vi "RT Main v0.96.vi"() -> ()   [LabVIEW 2017]
doc: "Changelog:\n\nv0.9:\n- Autocycle"
uses:
  Controls/Auto Delays.ctl
  support/Controls/All Inputs.ctl
  support/Controls/Index Details.ctl
  support/Controls/Auto Stats.ctl
  Controls/Auto Times.ctl
  Global Variables/RT GV.vi
  support/Message Queue/Enqueue Message (Single).vi
  Global Variables/FPGA GV.vi
  <vilib>/Utility/error.llb/Error Cluster From Error Code.vi
  <vilib>/rvi/errors/niLvFpgaAdjustHostInterfaceError.vi
  Global Variables/Network Globals.vi
  <vilib>/FPGAPlugInAG/Dynamic/niLvFpga_Close_Dynamic.vi
  <vilib>/rvi/interface/nirviReadWriteControl/nirviReadWriteControl.xnode
  Controls/FPGA Ref.ctl
  <vilib>/rvi/interface/nirviCloseFPGA/nirviCloseFPGA.xnode
  support/Message Queue/Message Queue.lvlib
  NiFpgaLv.dll
  <vilib>/rvi/interface/Simulation/niFpgaSimulationCallBeginRW.vi
panel:
  in  "Auto Para":T1={"Agitator Delays"=[250, 350], "TF Delays"=[700, 800, 2], "Insertion Delays"=[100, 500], "Cutting Delays"=[300, 300, 100], "PF Delays"=[250, 30000], "Measur. Delays"=[500.0, 188.9, 1.0], "Reject Delays"=[500], "BF Delays"=[1000, 1000]}
  in  "Counts in":cluster{"OutputCount":u32, "RejectCount":u32}
  in  "Stop Button 4":bool
  out "error out":errorcluster
  out "Wrong Message":string
  in  "Stop Button":bool
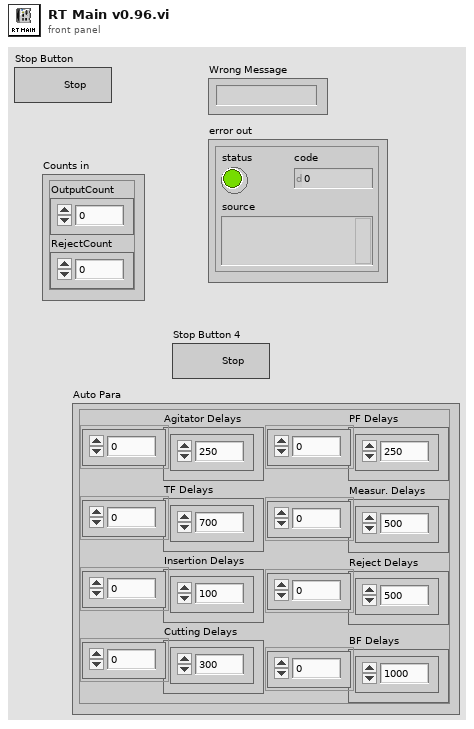
[diagram p1: front panel]
types:
  T1 = typedef "Auto Delays.ctl" = cluster{"Agitator Delays":u32[], "TF Delays":u32[], "Insertion Delays":u32[], "Cutting Delays":u32[], "PF Delays":u32[], "Measur. Delays":dbl[], "Reject Delays":u32[], "BF Delays":u32[]}
  T2 = typedef "FPGA Ref.ctl" = refnum<k20>
  T3 = cluster{"TL_Red":bool, "TL_Orange":bool, "TL_Green":bool, "TL_Buzzer":bool, "SOL_Index_Rotary_CW":bool, "SOL_Index_CNVR_Rotary_CCW":bool, "SOL_Index_CNVR_Stopper_Rear":bool, "SOL_Index_CNVR_Output _Separator _Rear":bool, "Bowl  Feeder_ ON":bool, "Pump_CNVR_Motor _ON":bool, "SOL_Gating_CYL_Rear":bool, "SOL_Tube_Feed_Agitatator":bool, "SOL_Tube_Feed_Gating_CYL":bool, "SOL_Insertion _CYL":bool, "SOL_Insertion_Clamp_CYL":bool, "SOL_Cutting_CYL":bool, "SOL_Cutting_Clamp_CYL":bool, "SOL_Insertion_Air_Nozzle":bool, "SOL_Measurement_CYL":bool, "SOL_Measure_Clamp_CYL":bool, "SOL_Rejection CYL_1":bool, "SOL_Rejection CYL_2":bool, "SOL_Rejection CYL_3":bool, "SOL_Rejection CYL_4":bool, "DO1.24":bool, "DO1.25":bool, "DO1.26":bool, "DO1.27":bool, "DO1.28":bool, "DO1.29":bool, "DO1.30":bool, "DO1.31":bool}
  T4 = typedef "All Inputs.ctl" = cluster{"DI 1":cluster{"Machine_ON":bool, "E_stop ":bool, "SW_Pressure":bool, "SW_Start ":bool, "SW_Reset":bool, "SW_Stop":bool, "SW_Door":bool, "RS_Index_Rotary_CW":bool, "RS_Index_Rotary_CCW":bool, "RS_Index_Stopper _Rear":bool, "RS_Index_Output_Separator_Rear":bool, "PES_Index_Pallet_Sensor":bool, "PES_Index_Output_Part Sensor":bool, "ICS_BF_Low_Level_1":bool, "ICS_BF_Low_Level_2":bool, "ICS_BF_Pump_CNVR_Full_1":bool, "ICS_BF_Pump_CNVR_Full_2":bool, "ICS_BF_Pump_CNVR_Full_3":bool, "ICS_BF_Pump_CNVR_Full_4":bool, "PES_PC_Pump Presence_1":bool, "PES_PC_Pump Presence_2":bool, "PES_PC_Pump Presence_3":bool, "PES_PC_Pump Presence_4":bool, "RS_PC_Gating_Front":bool, "PES_Pump_Interference":bool, "PES_TF_Low_Level":bool, "PES_Tube Presence_1":bool, "PES_Tube Presence_2":bool, "PES_Tube Presence_3":bool, "PES_Tube Presence_4":bool, "DI1.30":bool, "DI1.31":bool}, "DI 2":cluster{"RS_Agitatator_1_Rear ":bool, "RS_Agitatator_2_Rear ":bool, "RS_TF_Gating CYL_Rear":bool, "RS_Insertion_1_Rear":bool, "RS_Insertion_1_Front":bool, "RS_Insertion _2_Rear":bool, "RS_Insertion _2_Front":bool, "RS_Insertion _3_Rear":bool, "RS_Insertion _3_Front":bool, "RS_Insertion _4_Rear":bool, "RS_Insertion _4_Front":bool, "RS_Insertion_Clamp_Rear":bool, "RS_Cutting_Rear":bool, "RS_Cutting_Clamp _Rear":bool, "RS_Measurement_1_Rear":bool, "RS_Measurement_2_Rear":bool, "RS_Measurement_3_Rear":bool, "RS_Measurement_4_Rear":bool, "RS_Measure_Clamp_Rear":bool, "RS_Rejection_1_Rear":bool, "RS_Rejection_2_Rear":bool, "RS_Rejection_3_Rear":bool, "RS_Rejection_4_Rear":bool, "DI2.23":bool, "DI2.24":bool, "DI2.25":bool, "DI2.26":bool, "DI2.27":bool, "DI2.28":bool, "DI2.29":bool, "DI2.30":bool, "DI2.31":bool}, "IAS 1":dbl, "IAS 2":dbl, "IAS 3":dbl, "IAS 4":dbl, "DO 1":cluster{"TL_Red":bool, "TL_Orange":bool, "TL_Green":bool, "TL_Buzzer":bool, "SOL_Index_Rotary_CW":bool, "SOL_Index_CNVR_Rotary_CCW":bool, "SOL_Index_CNVR_Stopper_Rear":bool, "SOL_Index_CNVR_Output _Separator _Rear":bool, "Bowl  Feeder_ ON 1":bool, "Pump_CNVR_Motor _ON":bool, "SOL_PC_Gating_CYL_Rear":bool, "SOL_Tube_Feed_Agitatator":bool, "SOL_Tube_Feed_Gating_CYL":bool, "SOL_Insertion _CYL":bool, "SOL_Insertion_Clamp_CYL":bool, "SOL_Cutting_CYL":bool, "SOL_Cutting_Clamp_CYL":bool, "SOL_Insertion_Air_Nozzle":bool, "SOL_Measurement_CYL":bool, "DO1.19":bool, "SOL_Rejection CYL_1":bool, "SOL_Rejection CYL_2":bool, "SOL_Rejection CYL_3":bool, "SOL_Rejection CYL_4":bool, "Bowl  Feeder_ ON 2":bool, "SOL_BF_BlowerON":bool, "SOL_BF1_Track1":bool, "SOL_BF1_Track2":bool, "SOL_BF2_Track1":bool, "SOL_BF2_Track2":bool, "DO1.30":bool, "DO1.31":bool}}
  T5 = typedef "Index Details.ctl" = cluster{"Time (ms)":u32, "Waveform Graph":i16[]}
  T6 = cluster{T1, "Reject Pallets":cluster{"Reject 1":bool, "Reject 2":bool, "Reject 3":bool, "Reject 4":bool}}
  T7 = typedef "Auto Stats.ctl" = cluster{"Time":timestamp, "OEE":cluster{"AVL":dbl, "PRF":dbl, "QUA":dbl, "OEE":dbl}, "Auto Times":T8, "Counts out":cluster{"OutputCount":u32, "RejectCount":u32}, "Measurements":cluster{"1":dbl, "2":dbl, "3":dbl, "4":dbl}, "Outputs":cluster{"OutputCount":u32, "Numeric Control":u32}}
  T8 = typedef "Auto Times.ctl" = cluster{"Index Time":u32, "TF Time":u32, "Insertion Time":u32, "Cutting Time":u32, "PF Time":u32, "Meas. Time":u32, "Reject Time":u32}
  T9 = cluster{string, dbl, "Counts in":cluster{"OutputCount":u32, "RejectCount":u32}, "Auto Para":T1}
  T10 = cluster{"TL_Red":bool, "TL_Orange":bool, "TL_Green":bool, "TL_Buzzer":bool, "SOL_Index_Rotary_CW":bool, "SOL_Index_CNVR_Rotary_CCW":bool, "SOL_Index_CNVR_Stopper_Rear":bool, "SOL_Index_CNVR_Output _Separator _Rear":bool, "Bowl Feeder_ ON1":bool, "Pump_CNVR_Motor _ON":bool, "SOL_PC_Gating_CYL_Rear":bool, "SOL_Tube_Feed_Agitatator":bool, "SOL_Tube_Feed_Gating_CYL":bool, "SOL_Insertion _CYL":bool, "SOL_Insertion_Clamp_CYL":bool, "SOL_Cutting_CYL":bool, "SOL_Cutting_Clamp_CYL":bool, "SOL_Insertion_Air_Nozzle":bool, "SOL_Measurement_CYL":bool, "DO1.19":bool, "SOL_Rejection CYL_1":bool, "SOL_Rejection CYL_2":bool, "SOL_Rejection CYL_3":bool, "SOL_Rejection CYL_4":bool, "Bowl Feeder_ON2":bool, "SOL_BF_BlowerON":bool, "SOL_BF1_Track1":bool, "SOL_BF1_Track2":bool, "SOL_BF2_Track1":bool, "SOL_BF2_Track2":bool, "DO1.30":bool, "DO1.31":bool}
  T11 = cluster{"Machine_ON":bool, "E_stop ":bool, "SW_Pressure":bool, "SW_Start ":bool, "SW_Reset":bool, "SW_Stop":bool, "SW_Door":bool, "RS_Index_Rotary_CW":bool, "RS_Index_Rotary_CCW":bool, "RS_Index_Stopper _Rear":bool, "RS_Index_Output_Separator_Rear":bool, "PES_Index_Pallet_Sensor":bool, "PES_Index_Output_Part Sensor":bool, "ICS_BF_Low_Level_1":bool, "ICS_BF_Low_Level_2":bool, "ICS_BF_Pump_CNVR_Full_1":bool, "ICS_BF_Pump_CNVR_Full_2":bool, "ICS_BF_Pump_CNVR_Full_3":bool, "ICS_BF_Pump_CNVR_Full_4":bool, "PES_PC_Pump Presence_1":bool, "PES_PC_Pump Presence_2":bool, "PES_PC_Pump Presence_3":bool, "PES_PC_Pump Presence_4":bool, "RS_PC_Gating_Front":bool, "PES_Pump_Interference":bool, "PES_TF_Low_Level":bool, "PES_Tube Presence_1":bool, "PES_Tube Presence_2":bool, "PES_Tube Presence_3":bool, "PES_Tube Presence_4":bool, "DI1.30":bool, "DI1.31":bool}
  T12 = cluster{"RS_Agitatator_1_Rear ":bool, "RS_Agitatator_2_Rear ":bool, "RS_TF_Gating CYL_Rear":bool, "RS_Insertion_1_Rear":bool, "RS_Insertion_1_Front":bool, "RS_Insertion _2_Rear":bool, "RS_Insertion _2_Front":bool, "RS_Insertion _3_Rear":bool, "RS_Insertion _3_Front":bool, "RS_Insertion _4_Rear":bool, "RS_Insertion _4_Front":bool, "RS_Insertion_Clamp_Rear":bool, "RS_Cutting_Rear":bool, "RS_Cutting_Clamp _Rear":bool, "RS_Measurement_1_Rear":bool, "RS_Measurement_2_Rear":bool, "RS_Measurement_3_Rear":bool, "RS_Measurement_4_Rear":bool, "DI2.18":bool, "RS_Rejection_1_Rear":bool, "RS_Rejection_2_Rear":bool, "RS_Rejection_3_Rear":bool, "RS_Rejection_4_Rear":bool, "DI2.23":bool, "DI2.24":bool, "DI2.25":bool, "DI2.26":bool, "DI2.27":bool, "DI2.28":bool, "DI2.29":bool, "DI2.30":bool, "DI2.31":bool}
  T13 = cluster{"Array":string[][], "Machine Status":string}
  T14 = cluster{"Measurements":cluster{"1":dbl, "2":dbl, "3":dbl, "4":dbl}, "Reject Pallets":cluster{"Reject 1":bool, "Reject 2":bool, "Reject 3":bool, "Reject 4":bool}}
  T15 = cluster{"Auto Times":T8, "Results":cluster{"Measurements":cluster{"1":dbl, "2":dbl, "3":dbl, "4":dbl}, "Reject Pallets":cluster{"Reject 1":bool, "Reject 2":bool, "Reject 3":bool, "Reject 4":bool}}, "OutputCount":u32, "error out":errorcluster}
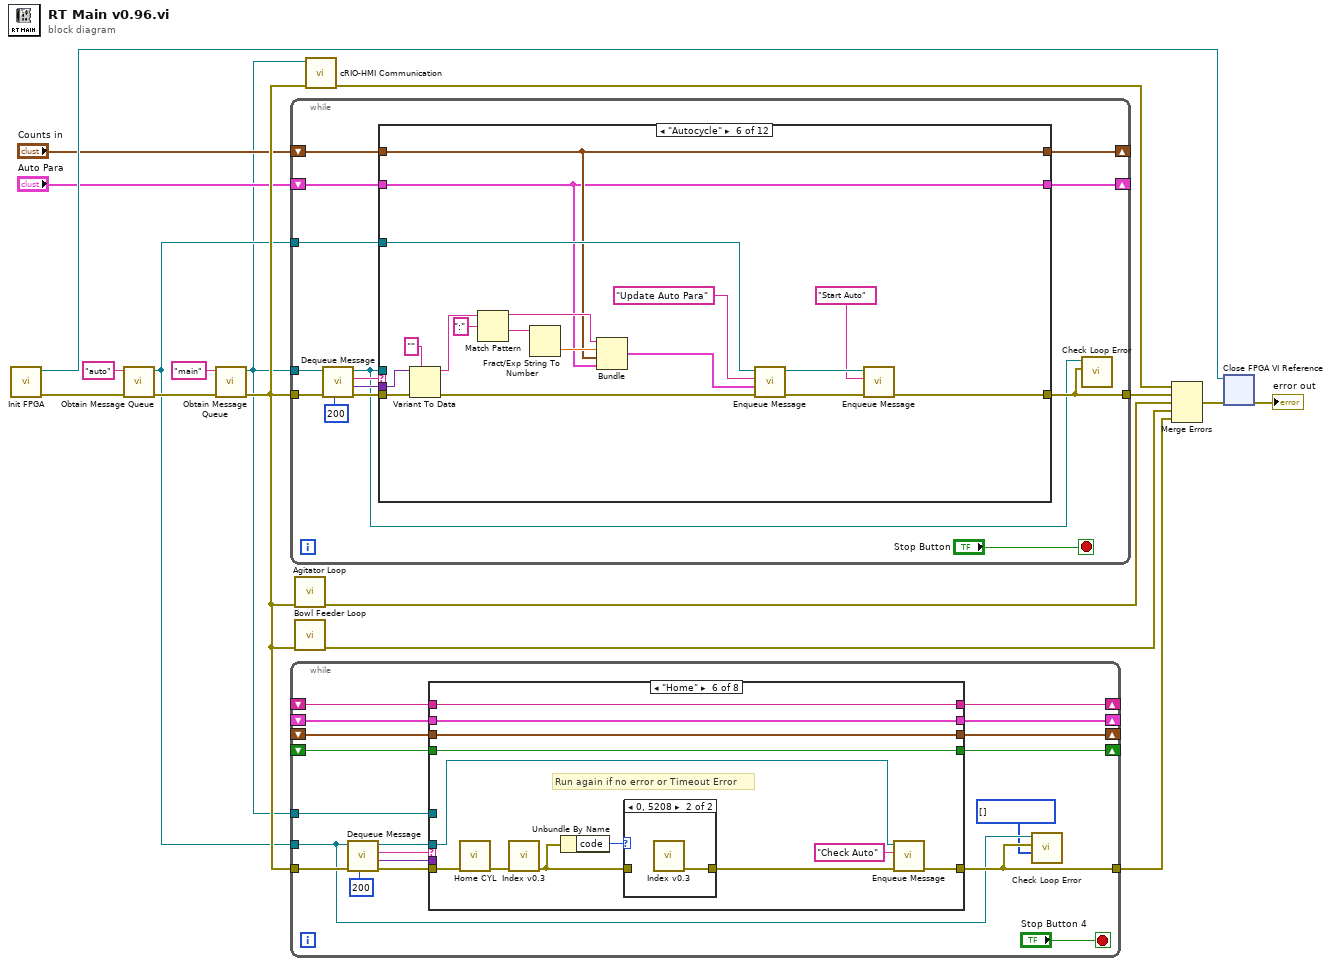
[diagram p0: block diagram]
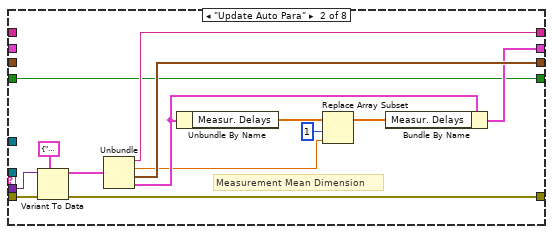
[diagram p3: hidden frame]
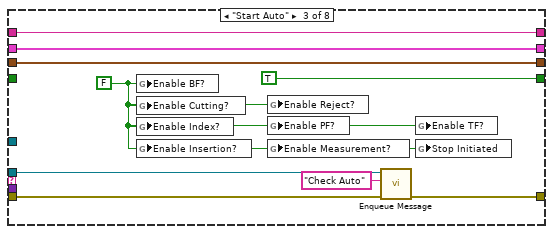
[diagram p4: hidden frame]
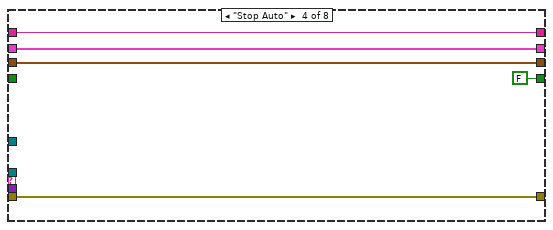
[diagram p5: hidden frame]
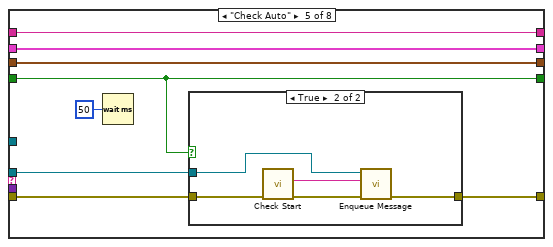
[diagram p6: hidden frame]
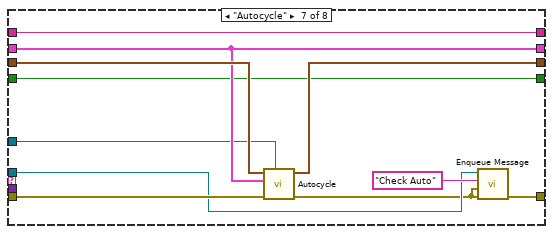
[diagram p9: hidden frame]
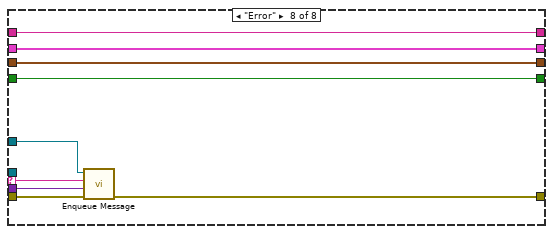
[diagram p10: hidden frame]
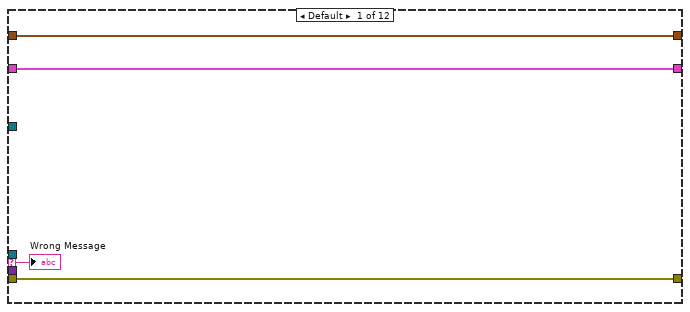
[diagram p11: hidden frame]
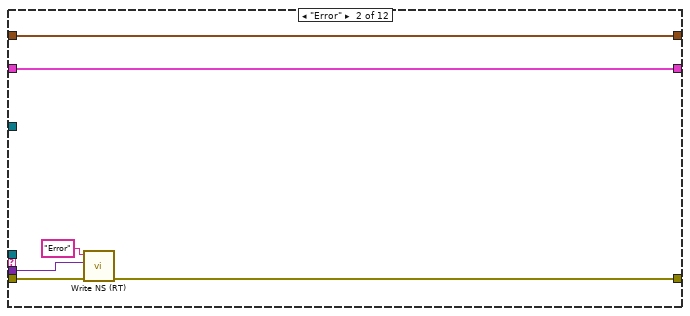
[diagram p12: hidden frame]
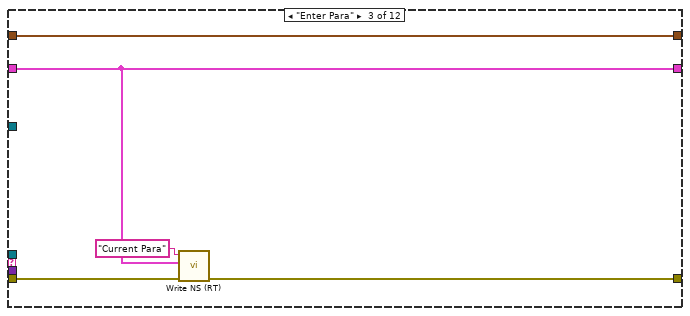
[diagram p13: hidden frame]
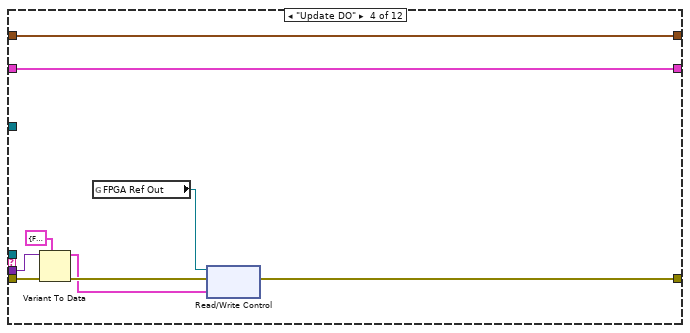
[diagram p14: hidden frame]
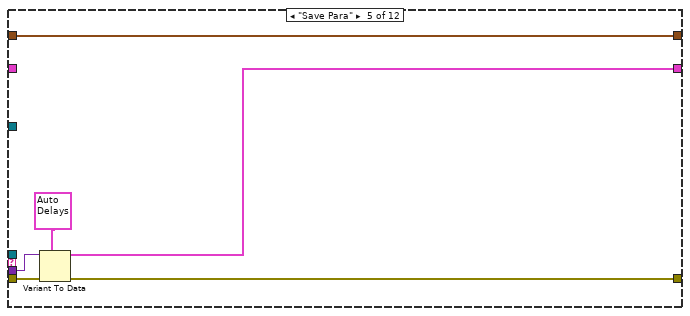
[diagram p15: hidden frame]
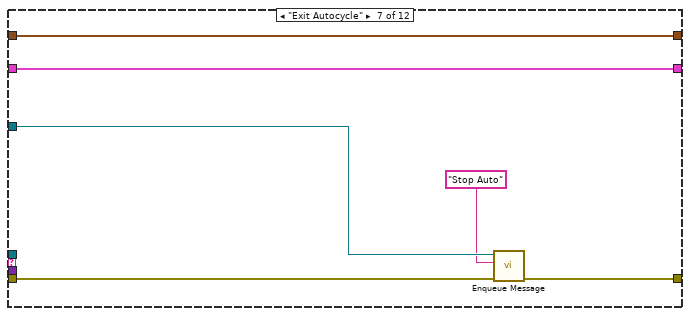
[diagram p16: hidden frame]
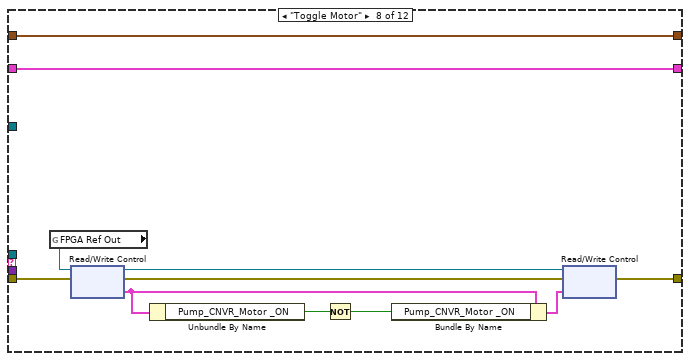
[diagram p17: hidden frame]
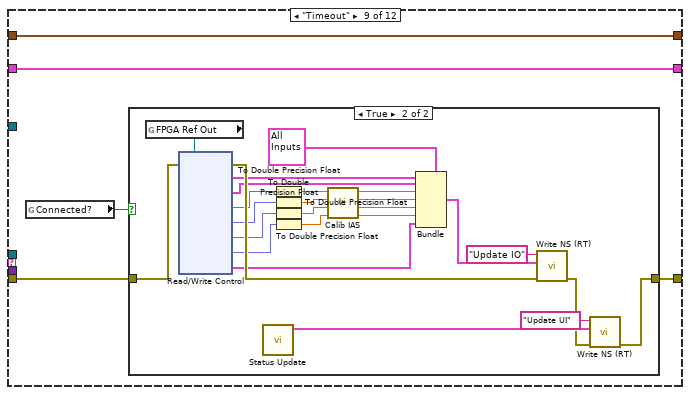
[diagram p18: hidden frame]
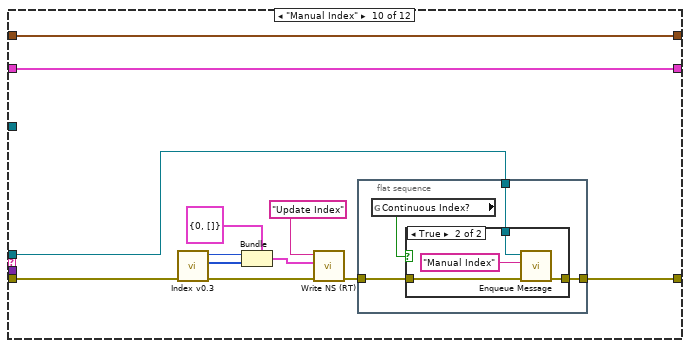
[diagram p20: hidden frame]
diagram:
  n1 = call "Init FPGA.vi"() -> ("error out"=w6:errorcluster, "FPGA Ref Out"=w11:T2)  [unwired: 10 in]
  n2 = call "Obtain Message Queue.vi"("error in (no error)"=w6, "name"="auto") -> ("error out"=w5:errorcluster, "Message Queue"=w2:refnum<queue>)  [unwired: 8 in]
  n3 = call "Obtain Message Queue.vi"("error in (no error)"=w5, "name"="main") -> ("error out"=w10:errorcluster, "Message Queue"=w1:refnum<queue>)  [unwired: 8 in]
  n4 = while {
    tunnel: w10 -> [w30]
    tunnel: w1 -> [w29]
    tunnel: [w25] -> w17
    tunnel: w2 -> [w22]
    shift-right: [w19] -> _
    shift-left: "Auto Para" -> [w20]
    shift-right: [w18] -> _
    shift-left: "Counts in" -> [w21]
    stop <- "Stop Button" stop-if-true
    n5 = call "Dequeue Message.vi"("timeout"=200, "error in (no error)"=w30, "Message Queue"=w29) -> ("error out"=w28:errorcluster, "Message Data"=w26:variant, "Message"=w27:string, "dup Message Queue"=w24:refnum<queue>)  [unwired: 5 in]
    n6 = case shown="\"Autocycle\"" w27 {
      selector: w27 -> [w35 _ _ _ _ _ _ _ _ _ _ _]
      tunnel: w28 -> [w34 w39 w46 w55 w61 w79 w85 w95 w100 w139 w166 w176]
      tunnel: w24 -> [_ _ _ _ _ _ _ _ _ w131 _ _]
      tunnel: w26 -> [_ w37 _ w54 w60 w78 _ _ _ _ w165 w175]
      tunnel: [w34 w38 w45 w50 w59 w64 w81 w93 w101 w132 w161 w172] -> w25
      tunnel: w22 -> [_ _ _ _ _ w71 w84 _ _ _ _ _]
      tunnel: w21 -> [w33 w41 w43 w48 w58 w68 w83 w87 w98 w128 w152 w171]
      tunnel: w20 -> [w32 w40 w42 w47 _ w67 w82 w86 w97 w129 w151 w170]
      tunnel: [w32 w40 w42 w47 w57 w67 w82 w86 w97 w129 w151 w170] -> w19
      tunnel: [w33 w41 w43 w48 w58 w68 w83 w87 w98 w128 w152 w171] -> w18
      frame Default {
        "Wrong Message" <- w35
      }
      frame "Error" {
        n7 = call "Write NS (RT).vi"("error in (no error)"=w39, "Message Data"=w37, "Message"="Error") -> ("error out"=w38:errorcluster)  [unwired: 8 in]
      }
      frame "Enter Para" {
        n8 = call "Write NS (RT).vi"("error in (no error)"=w46, "Message Data"=w42, "Message"="Current Para") -> ("error out"=w45:errorcluster)  [unwired: 8 in]
      }
      frame "Update DO" {
        n9 = Variant To Data(error in=w55, type=T3 {"TL_Red"=FALSE, "TL_Orange"=FALSE, "TL_Green"=FALSE, "TL_Buzzer"=FALSE, "SOL_Index_Rotary_CW"=FALSE, "SOL_Index_CNVR_Rotary_CCW"=FALSE, "SOL_Index_CNVR_Stopper_Rear"=FALSE, "SOL_Index_CNVR_Output _Separator _Rear"=FALSE, "Bowl  Feeder_ ON"=FALSE, "Pump_CNVR_Motor _ON"=FALSE, "SOL_Gating_CYL_Rear"=FALSE, "SOL_Tube_Feed_Agitatator"=FALSE, "SOL_Tube_Feed_Gating_CYL"=FALSE, "SOL_Insertion _CYL"=FALSE, "SOL_Insertion_Clamp_CYL"=FALSE, "SOL_Cutting_CYL"=FALSE, "SOL_Cutting_Clamp_CYL"=FALSE, "SOL_Insertion_Air_Nozzle"=FALSE, "SOL_Measurement_CYL"=FALSE, "SOL_Measure_Clamp_CYL"=FALSE, "SOL_Rejection CYL_1"=FALSE, "SOL_Rejection CYL_2"=FALSE, "SOL_Rejection CYL_3"=FALSE, "SOL_Rejection CYL_4"=FALSE, "DO1.24"=FALSE, "DO1.25"=FALSE, "DO1.26"=FALSE, "DO1.27"=FALSE, "DO1.28"=FALSE, "DO1.29"=FALSE, "DO1.30"=FALSE, "DO1.31"=FALSE} ("DO 1"), Variant=w54) -> (data=w49:T3, error out=w51:errorcluster)
        n10 = global read "FPGA GV.vi" "FPGA Ref Out"() -> (w52:T2)
        n11 = xnode "Read/Write Control"("FPGA VI Reference In"=w52, "error in"=w51, "DO 1"=w49) -> ("error out"=w50:errorcluster)  [unwired: 1 out]
      }
      frame "Save Para" {
        n12 = Variant To Data(error in=w61, type=T1 {"Agitator Delays"=[700, 250], "TF Delays"=[700, 800, 2], "Insertion Delays"=[100, 500], "Cutting Delays"=[300, 300, 100], "PF Delays"=[250, 30000], "Measur. Delays"=[500.0, 188.9, 1.0], "Reject Delays"=[500], "BF Delays"=[1000, 1000]} ("Auto Para"), Variant=w60) -> (data=w57:T1, error out=w59:errorcluster)
      }
      frame "Autocycle" {
        n13 = Variant To Data(error in=w79, type="", Variant=w78) -> (data=w74:string, error out=w72:errorcluster)
        n14 = Match Pattern(string=w74, regular expression=":") -> (before substring=w70:string, after substring=w75:string)  [unwired: 1 in, 2 out]
        n15 = Fract/Exp String To Number(string=w75) -> (number=w69:dbl)  [unwired: 3 in, 1 out]
        n16 = Bundle(w70, w69, "Counts in"=w68, "Auto Para"=w67) -> (w66:T9)  [unwired: 1 in]
        n17 = call-poly "Enqueue Message.vi"("error in (no error)"=w72, "Message Data"=w66, "Message"="Update Auto Para", "Message Queue"=w71) -> ("error out"=w65:errorcluster, "dup Message Queue"=w63:refnum<queue>)  [unwired: 6 in]
        n18 = call-poly "Enqueue Message.vi"("error in (no error)"=w65, "Message"="Start Auto", "Message Queue"=w63) -> ("error out"=w64:errorcluster)  [unwired: 7 in, 1 out]
      }
      frame "Exit Autocycle" {
        n19 = call-poly "Enqueue Message.vi"("error in (no error)"=w85, "Message"="Stop Auto", "Message Queue"=w84) -> ("error out"=w81:errorcluster)  [unwired: 7 in, 1 out]
      }
      frame "Toggle Motor" {
        n20 = global read "FPGA GV.vi" "FPGA Ref Out"() -> (w96:T2)
        n21 = xnode "Read/Write Control"("FPGA VI Reference In"=w96, "error in"=w95) -> ("FPGA VI Reference Out"=w92:T2, "error out"=w94:errorcluster, "DO 1"=w90:T10)
        n22 = Unbundle By Name(w90) -> ("Pump_CNVR_Motor _ON"=w91:bool)
        n23 = Not(x=w91) -> (.not. x?=w88:bool)
        n24 = Bundle By Name(cluster=w90, "Pump_CNVR_Motor _ON"=w88) -> (w89:T10)
        n25 = xnode "Read/Write Control"("FPGA VI Reference In"=w92, "error in"=w94, "DO 1"=w89) -> ("error out"=w93:errorcluster)  [unwired: 1 out]
      }
      frame "Timeout" {
        n26 = global read "Network Globals.vi" "Connected?"() -> (w99:bool)
        n27 = case shown="True" w99 {
          tunnel: [w102 w104] -> w101
          tunnel: w100 -> [w102 w126]
          frame False {
          }
          frame True {
            n28 = global read "FPGA GV.vi" "FPGA Ref Out"() -> (w103:T2)
            n29 = xnode "Read/Write Control"("FPGA VI Reference In"=w103, "error in"=w126) -> ("error out"=w125:errorcluster, "DI 1"=w124:T11, "DI 2"=w123:T12, "AI0"=w122:fxp<+/-,27,6>, "AI1"=w121:fxp<+/-,27,6>, "AI2"=w120:fxp<+/-,27,6>, "AI3"=w119:fxp<+/-,27,6>, "DO 1"=w116:T10)  [unwired: 1 out]
            n30 = call "Status Update.vi"() -> ("Status Cluster"=w106:T13)  [unwired: 11 in]
            n31 = To Double Precision Float(number=w122) -> (double precision float=w109:dbl)
            n32 = To Double Precision Float(number=w121) -> (double precision float=w111:dbl)
            n33 = To Double Precision Float(number=w120) -> (double precision float=w113:dbl)
            n34 = To Double Precision Float(number=w119) -> (double precision float=w115:dbl)
            n35 = call "Calib IAS.vi"("x 4"=w115, "x 3"=w113, "x 2"=w111, "x"=w109) -> ("y 4"=w114:dbl, "y 3"=w112:dbl, "y 2"=w110:dbl, "y 1"=w108:dbl)  [unwired: 4 in]
            n36 = Bundle(cluster=T4 {"DI 1"={"Machine_ON"=FALSE, "E_stop "=FALSE, "SW_Pressure"=FALSE, "SW_Start "=FALSE, "SW_Reset"=FALSE, "SW_Stop"=FALSE, "SW_Door"=FALSE, "RS_Index_Rotary_CW"=FALSE, "RS_Index_Rotary_CCW"=FALSE, "RS_Index_Stopper _Rear"=FALSE, "RS_Index_Output_Separator_Rear"=FALSE, "PES_Index_Pallet_Sensor"=FALSE, "PES_Index_Output_Part Sensor"=FALSE, "ICS_BF_Low_Level_1"=FALSE, "ICS_BF_Low_Level_2"=FALSE, "ICS_BF_Pump_CNVR_Full_1"=FALSE, "ICS_BF_Pump_CNVR_Full_2"=FALSE, "ICS_BF_Pump_CNVR_Full_3"=FALSE, "ICS_BF_Pump_CNVR_Full_4"=FALSE, "PES_PC_Pump Presence_1"=FALSE, "PES_PC_Pump Presence_2"=FALSE, "PES_PC_Pump Presence_3"=FALSE, "PES_PC_Pump Presence_4"=FALSE, "RS_PC_Gating_Front"=FALSE, "PES_Pump_Interference"=FALSE, "PES_TF_Low_Level"=FALSE, "PES_Tube Presence_1"=FALSE, "PES_Tube Presence_2"=FALSE, "PES_Tube Presence_3"=FALSE, "PES_Tube Presence_4"=FALSE, "DI1.30"=FALSE, "DI1.31"=FALSE}, "DI 2"={"RS_Agitatator_1_Rear "=FALSE, "RS_Agitatator_2_Rear "=FALSE, "RS_TF_Gating CYL_Rear"=FALSE, "RS_Insertion_1_Rear"=FALSE, "RS_Insertion_1_Front"=FALSE, "RS_Insertion _2_Rear"=FALSE, "RS_Insertion _2_Front"=FALSE, "RS_Insertion _3_Rear"=FALSE, "RS_Insertion _3_Front"=FALSE, "RS_Insertion _4_Rear"=FALSE, "RS_Insertion _4_Front"=FALSE, "RS_Insertion_Clamp_Rear"=FALSE, "RS_Cutting_Rear"=FALSE, "RS_Cutting_Clamp _Rear"=FALSE, "RS_Measurement_1_Rear"=FALSE, "RS_Measurement_2_Rear"=FALSE, "RS_Measurement_3_Rear"=FALSE, "RS_Measurement_4_Rear"=FALSE, "RS_Measure_Clamp_Rear"=FALSE, "RS_Rejection_1_Rear"=FALSE, "RS_Rejection_2_Rear"=FALSE, "RS_Rejection_3_Rear"=FALSE, "RS_Rejection_4_Rear"=FALSE, "DI2.23"=FALSE, "DI2.24"=FALSE, "DI2.25"=FALSE, "DI2.26"=FALSE, "DI2.27"=FALSE, "DI2.28"=FALSE, "DI2.29"=FALSE, "DI2.30"=FALSE, "DI2.31"=FALSE}, "IAS 1"=0.0, "IAS 2"=0.0, "IAS 3"=0.0, "IAS 4"=0.0, "DO 1"={"TL_Red"=FALSE, "TL_Orange"=FALSE, "TL_Green"=FALSE, "TL_Buzzer"=FALSE, "SOL_Index_Rotary_CW"=FALSE, "SOL_Index_CNVR_Rotary_CCW"=FALSE, "SOL_Index_CNVR_Stopper_Rear"=FALSE, "SOL_Index_CNVR_Output _Separator _Rear"=FALSE, "Bowl  Feeder_ ON 1"=FALSE, "Pump_CNVR_Motor _ON"=FALSE, "SOL_PC_Gating_CYL_Rear"=FALSE, "SOL_Tube_Feed_Agitatator"=FALSE, "SOL_Tube_Feed_Gating_CYL"=FALSE, "SOL_Insertion _CYL"=FALSE, "SOL_Insertion_Clamp_CYL"=FALSE, "SOL_Cutting_CYL"=FALSE, "SOL_Cutting_Clamp_CYL"=FALSE, "SOL_Insertion_Air_Nozzle"=FALSE, "SOL_Measurement_CYL"=FALSE, "DO1.19"=FALSE, "SOL_Rejection CYL_1"=FALSE, "SOL_Rejection CYL_2"=FALSE, "SOL_Rejection CYL_3"=FALSE, "SOL_Rejection CYL_4"=FALSE, "Bowl  Feeder_ ON 2"=FALSE, "SOL_BF_BlowerON"=FALSE, "SOL_BF1_Track1"=FALSE, "SOL_BF1_Track2"=FALSE, "SOL_BF2_Track1"=FALSE, "SOL_BF2_Track2"=FALSE, "DO1.30"=FALSE, "DO1.31"=FALSE}}, "DI 1"=w124, "DI 2"=w123, "IAS 1"=w108, "IAS 2"=w110, "IAS 3"=w112, "IAS 4"=w114, "DO 1"=w116) -> (w118:T4)
            n37 = call "Write NS (RT).vi"("error in (no error)"=w125, "Message Data"=w118, "Message"="Update IO") -> ("error out"=w105:errorcluster)  [unwired: 8 in]
            n38 = call "Write NS (RT).vi"("error in (no error)"=w105, "Message Data"=w106, "Message"="Update UI") -> ("error out"=w104:errorcluster)  [unwired: 8 in]
          }
        }
      }
      frame "Manual Index" {
        n39 = call "Index v0.3.vi"("error in (no error)"=w139) -> ("error out"=w137:errorcluster, "Waveform Graph"=w135:i16[], "Index Time"=w136:u32)  [unwired: 7 in, 1 out]
        n40 = Bundle(cluster=T5 {"Time (ms)"=0, "Waveform Graph"=[]}, "Time (ms)"=w136, "Waveform Graph"=w135) -> (w134:T5)
        n41 = call "Write NS (RT).vi"("error in (no error)"=w137, "Message Data"=w134, "Message"="Update Index") -> ("error out"=w133:errorcluster)  [unwired: 8 in]
        n42 = flat-sequence {
          tunnel: w133 -> [w143]
          tunnel: [w142] -> w132
          tunnel: w131 -> [w140]
          frame #0 {
            n43 = global read "RT GV.vi" "Continuous Index?"() -> (w141:bool)
            n44 = case shown="True" w141 {
              tunnel: w143 -> [w144 w148]
              tunnel: [w144 w147] -> w142
              tunnel: w140 -> [_ w145]
              frame False {
              }
              frame True {
                n45 = call-poly "Enqueue Message.vi"("error in (no error)"=w148, "Message"="Manual Index", "Message Queue"=w145) -> ("error out"=w147:errorcluster)  [unwired: 7 in, 1 out]
              }
            }
          }
        }
      }
      frame "Manual Run" {
        n46 = Variant To Data(error in=w166, type=T6 {{"Agitator Delays"=[1000], "TF Delays"=[1000], "Insertion Delays"=[1000], "Cutting Delays"=[1000], "PF Delays"=[1000], "Measur. Delays"=[1000.0], "Reject Delays"=[1000], "BF Delays"=[1000]}, "Reject Pallets"={"Reject 1"=FALSE, "Reject 2"=FALSE, "Reject 3"=FALSE, "Reject 4"=FALSE}}, Variant=w165) -> (data=w157:T6, error out=w164:errorcluster)
        n47 = Unbundle(w157) -> (w154:T1)  [unwired: 1 out]
        n48 = Unbundle By Name(w154) -> ("Agitator Delays"=w150:u32[], "BF Delays"=w149:u32[])
        n49 = call "Manual.vi"("error in"=w164, "Auto Delays"=w154) -> ("error out"=w156:errorcluster, "OutputCount"=w155:u32, "Results"=w153:T14, "Auto Times"=w160:T8)  [unwired: 6 in]
        n50 = global write "RT GV.vi" "Agitator Delays"(w150) -> ()
        n51 = global write "RT GV.vi" "BF Delays"(w149) -> ()
        n52 = Bundle("Auto Times"=w160, "Results"=w153, "OutputCount"=w155, "error out"=w156) -> (w159:T15)  [unwired: 1 in]
        n53 = call "Write NS (RT).vi"("Message Data"=w159, "Message"="Manual Status") -> ("error out"=w162:errorcluster)  [unwired: 9 in]
        n54 = Merge Errors(w162) -> (w161:errorcluster)
      }
      frame "Log Cycle" {
        n55 = Variant To Data(error in=w176, type=T7 {"Time"=timestamp(0 s since 1904-01-01), "OEE"={"AVL"=100.0, "PRF"=100.0, "QUA"=100.0, "OEE"=0.0}, "Auto Times"={"Index Time"=0, "TF Time"=0, "Insertion Time"=0, "Cutting Time"=0, "PF Time"=0, "Meas. Time"=0, "Reject Time"=0}, "Counts out"={"OutputCount"=0, "RejectCount"=0}, "Measurements"={"1"=0.0, "2"=0.0, "3"=0.0, "4"=0.0}, "Outputs"={"OutputCount"=0, "Numeric Control"=0}} ("Auto Stats"), Variant=w175) -> (data=w167:T7, error out=w168:errorcluster)
        n56 = call "Write NS (RT).vi"("error in (no error)"=w168, "Message Data"=w167, "Message"="Autocycle Log") -> ("error out"=w173:errorcluster)  [unwired: 8 in]
        n57 = Merge Errors(w173) -> (w172:errorcluster)
      }
    }
    n58 = call "Check Loop Error.vi"("error to process"=w25, "Message Queue"=w24) -> ()  [unwired: 8 in, 2 out]
  }
  n59 = while {
    tunnel: w10 -> [w191]
    tunnel: [w189] -> w9
    shift-right: [w193] -> _
    shift-left: _ -> [w194]
    tunnel: w2 -> [w181]
    shift-right: [w185] -> _
    shift-left: _ -> [w184]
    shift-right: [w183] -> _
    shift-left: _ -> [w182]
    shift-right: [w180] -> _
    shift-left: _ -> [w179]
    tunnel: w1 -> [w178]
    stop <- "Stop Button 4" stop-if-true
    n60 = call "Dequeue Message.vi"("timeout"=200, "error in (no error)"=w191, "Message Queue"=w181) -> ("error out"=w190:errorcluster, "Message Data"=w186:variant, "Message"=w187:string, "dup Message Queue"=w188:refnum<queue>)  [unwired: 5 in]
    n61 = case shown="\"Home\"" w187 {
      selector: w187 -> [_ _ _ _ _ _ _ w272]
      tunnel: w190 -> [w200 w214 w219 w225 w229 w250 w267 w270]
      tunnel: [w200 w213 w218 w225 w233 w245 w259 w269] -> w189
      tunnel: w194 -> [w199 _ w223 w228 w236 w254 w266 w276]
      tunnel: [w199 w208 w223 w228 w236 w254 w265 w276] -> w193
      tunnel: w188 -> [_ _ w217 _ w232 w243 w258 _]
      tunnel: w186 -> [_ w212 _ _ _ _ _ w271]
      tunnel: [w198 w209 w222 w227 w235 w253 w264 w275] -> w185
      tunnel: w184 -> [w198 _ w222 w227 w235 w253 w264 w275]
      tunnel: [w197 w202 w221 w226 w234 w252 w263 w274] -> w183
      tunnel: w182 -> [w197 _ w221 w226 w234 w252 w263 w274]
      tunnel: [w196 w201 TRUE FALSE w231 w251 w261 w273] -> w180
      tunnel: w179 -> [w196 w201 _ _ w231 w251 w261 w273]
      tunnel: w178 -> [_ _ _ _ _ _ w262 w268]
      frame Default {
      }
      frame "Update Auto Para" {
        # "Measurement Mean Dimension"
        n62 = Variant To Data(error in=w214, type=T9 {"", 0.0, "Counts in"={"OutputCount"=0, "RejectCount"=0}, "Auto Para"={"Agitator Delays"=[], "TF Delays"=[], "Insertion Delays"=[], "Cutting Delays"=[], "PF Delays"=[], "Measur. Delays"=[], "Reject Delays"=[], "BF Delays"=[]}} ("cluster"), Variant=w212) -> (data=w210:T9, error out=w213:errorcluster)
        n63 = Unbundle(w210) -> (w209:string, w204:dbl, "Counts in"=w208:cluster{"OutputCount":u32, "RejectCount":u32}, "Auto Para"=w207:T1)
        n64 = Unbundle By Name(w207) -> ("Measur. Delays"=w206:dbl[])
        n65 = Replace Array Subset(array=w206, new element=w204, index=1) -> (w203:dbl[])
        n66 = Bundle By Name(cluster=w207, "Measur. Delays"=w203) -> (w202:T1)
      }
      frame "Start Auto" {
        w215 = FALSE ("Enable BF?")
        n67 = global write "RT GV.vi" "Enable BF?"(w215) -> ()
        n68 = global write "RT GV.vi" "Enable Cutting?"(w215) -> ()
        n69 = global write "RT GV.vi" "Enable Index?"(w215) -> ()
        n70 = global write "RT GV.vi" "Enable Insertion?"(w215) -> ()
        n71 = global write "RT GV.vi" "Enable Reject?"(w215) -> ()
        n72 = global write "RT GV.vi" "Enable PF?"(w215) -> ()
        n73 = global write "RT GV.vi" "Enable Measurement?"(w215) -> ()
        n74 = call-poly "Enqueue Message.vi"("error in (no error)"=w219, "Message"="Check Auto", "Message Queue"=w217) -> ("error out"=w218:errorcluster)  [unwired: 7 in, 1 out]
        n75 = global write "RT GV.vi" "Enable TF?"(w215) -> ()
        n76 = global write "RT GV.vi" "Stop Initiated"(w215) -> ()
      }
      frame "Stop Auto" {
      }
      frame "Check Auto" {
        n77 = Wait (ms)(milliseconds to wait=u32 50) -> ()  [unwired: 1 out]
        n78 = case shown="True" w231 {
          tunnel: [w237 w242] -> w233
          tunnel: w232 -> [_ w238]
          tunnel: w229 -> [w237 w241]
          frame False {
          }
          frame True {
            n79 = call "Check Start.vi"("error in"=w241) -> ("error out"=w240:errorcluster, "Message"=w239:string)  [unwired: 9 in]
            n80 = call-poly "Enqueue Message.vi"("error in (no error)"=w240, "Message"=w239, "Message Queue"=w238) -> ("error out"=w242:errorcluster)  [unwired: 7 in, 1 out]
          }
        }
      }
      frame "Home" {
        # "Run again if no error or Timeout Error"
        n81 = call "Home CYL.vi"("error in"=w250) -> ("error out"=w249:errorcluster)  [unwired: 10 in]
        n82 = call "Index v0.3.vi"("error in (no error)"=w249) -> ("error out"=w247:errorcluster)  [unwired: 7 in, 3 out]
        n83 = Unbundle By Name(w247) -> ("code"=w248:i32)
        n84 = case shown="0, 5208" w248 {
          tunnel: [w255 w256] -> w244
          tunnel: w247 -> [w255 _]
          frame Default {
          }
          frame 0, 5208 {
            n85 = call "Index v0.3.vi"() -> ("error out"=w256:errorcluster)  [unwired: 8 in, 3 out]
          }
        }
        n86 = call-poly "Enqueue Message.vi"("error in (no error)"=w244, "Message"="Check Auto", "Message Queue"=w243) -> ("error out"=w245:errorcluster)  [unwired: 7 in, 1 out]
      }
      frame "Autocycle" {
        n87 = call "Autocycle.vi"("Message Queue"=w262, "error in"=w267, "Auto Para"=w263, "Counts in"=w266) -> ("error out"=w257:errorcluster, "Counts out"=w265:cluster{"OutputCount":u32, "RejectCount":u32})  [unwired: 6 in]
        n88 = call-poly "Enqueue Message.vi"("error in (no error)"=w257, "Message Data"=w257, "Message"="Check Auto", "Message Queue"=w258) -> ("error out"=w259:errorcluster)  [unwired: 6 in, 1 out]
      }
      frame "Error" {
        n89 = call-poly "Enqueue Message.vi"("error in (no error)"=w270, "Message Data"=w271, "Message"=w272, "Message Queue"=w268) -> ("error out"=w269:errorcluster)  [unwired: 6 in, 1 out]
      }
    }
    n90 = call "Check Loop Error.vi"("Ignore Errors"=i32[] [], "error to process"=w189, "Message Queue"=w181) -> ()  [unwired: 7 in, 2 out]
  }
  n91 = call "Agitator Loop.vi"("error in (no error)"=w10) -> ("error out"=w13:errorcluster)  [unwired: 10 in]
  n92 = call "Bowl Feeder Loop.vi"("error in (no error)"=w10) -> ("error out"=w12:errorcluster)  [unwired: 10 in]
  n93 = call "cRIO-HMI Communication.vi"("error in (no error)"=w10, "Message Queue"=w1) -> ("error out"=w16:errorcluster)  [unwired: 9 in]
  n94 = Merge Errors(w16, w17, w13, w12, w9) -> (w15:errorcluster)
  n95 = xnode ("Close FPGA VI Reference")("FPGA VI Reference In"=w11, "error in"=w15) -> ("error out"=→"error out":errorcluster)
